vi "SVO.vi"(0 "System no.":i32=1 min=1 max=4 step=1, 2 "Axes to command":string[](array[string]), 3 "Servo mode":bool[](array[boolean]), 5 "error in":errorcluster, 6 "Without axis ID?":bool) -> (19 "error out":errorcluster)   [LabVIEW 2026]
doc: "GCS 3.0\n=====\n\nSVO (Set Servo Mode)\n\nDescription\nSVO sets the mode of operation of the axis by specifying the values 0 or 1 as follows:\n0 -> 0x1 Open-Loop Position\n1 -> 0x2 Closed-Loop Position \nThe mode of operation can only be set when the axis is in the Operation enabled state. For \nfurther details, see \"Drive State Machine\" (p. 101). \n\nFormat\nSVO <AxisID> <Value>\n\nArguments\n<AxisID>\nAn axis of the controller\nThe available axes can be queried with USG? SYS.\nPossible values: Alias of the axis (p. 94) \n<Value>\nValue that sets the mode of operation of the axis\nPossible values:\n0 -> 0x1 Open-Loop Position\n1 -> 0x2 Closed-Loop Position\n\nResponse\nnone\n\nExample\nAxis 1 is to be operated in position control.\n>>svo?\n<<AXIS_1=0\n<<AXIS_2=0\n>>sam?\n<<AXIS_1=0x0\n<<AXIS_2=0x0\n>>svo axis_1 1\n>>svo?\n<<AXIS_1=1\n<<AXIS_2=0\n>>sam?\n<<AXIS_1=0x2\n<<AXIS_2=0x0\n\nNotes\nWith the SVO? command (p. 68), it can be queried whether the current mode of operation is \n0x2.\nThe mode of operation is also displayed in the status register of the axis, which can be queried \nwith the STV? command (p. 66). \nThe SAM command (p. 52) can be used to set all modes of operation supported for the axis.\n\nUser command level\nUSR\n\n\nGCS 2.0\n=====\n\nSets servo-control mode for given axes. If Without axis ID is TRUE, then Axes to command is ignored and first field of Servo mode array is used.\n\nE-516, E-517, E-518: Make sure that all servo switches on the piezo control electronics are set to \"Off\" to give the interface/display module complete control over the servo state.\n\nE-755: Without axis ID = FALSE. When the servo mode is switched off, RNP is automatically performed for the corresponding Nexline channel, which could take a few seconds. Command not available for E-755.101.\n\nE-816: Without axis ID = FALSE. Only one axis per command allowed.\n\nE-861: If you have enabled servo controller is busy for 100 ms, only after this period a next command can be performed.\n\nC-887, F-206, M-8X0: For GCS syntax version = GCS 2.0 or higher (check with CSV?.vi. If CSV?.vi is not supported, syntax version is GCS 1.0), Without axis ID = FALSE. For GCS 1.0, Without axis ID = TRUE and only first field of Servo mode array is valid. \n\nAll other systems: Without axis ID = FALSE"
panel:
  # "SVO (Set Servo Mode)\n\nSVO sets the mode of operation of the axis by specifying the values 0 or 1 as follows:\n0 -> 0x1 Open-Loop Position\n1 -> 0x2 Closed-Loop Position \nThe mode of operation can only be set when the axis is in the Operation enabled state. For \nfurther details, see \"Drive State Machine\"."
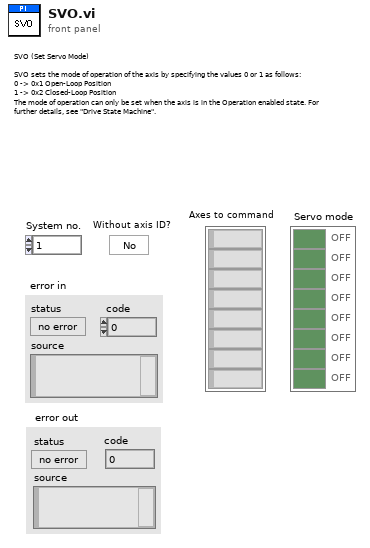
[diagram p1: front panel]
types:
  T1 = typedef "Syntax.ctl" = enum16{"GCS 1.0", "GCS 2.0", "GCS 3.0"}
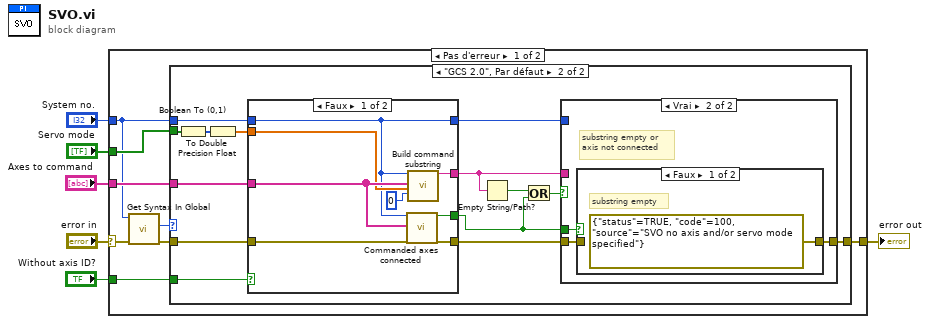
[diagram p0: block diagram]
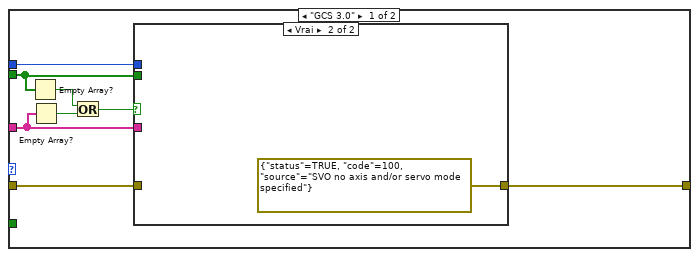
[diagram p2: hidden frame]
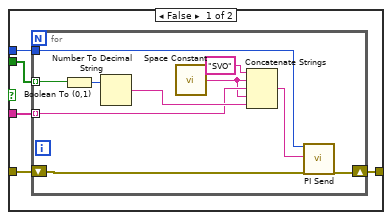
[diagram p3: hidden frame]
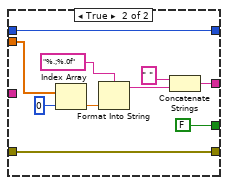
[diagram p4: hidden frame]
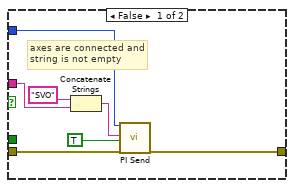
[diagram p5: hidden frame]
diagram:
  n1 = case shown="Pas d'erreur" "error in" {
    selector: "error in" -> [w10 w83]
    tunnel: [w14 w83] -> w6
    tunnel: "System no." -> [w7 _]
    tunnel: "Axes to command" -> [w13 _]
    tunnel: "Servo mode" -> [w12 _]
    tunnel: "Without axis ID?" -> [w11 _]
    frame No Error {
      n2 = call "Get Syntax In Global.vi"("error in"=w10, "System no."=w7) -> ("error out"=w9:errorcluster, "Syntax"=w8:T1)  [unwired: 8 in]
      n3 = case shown="\"GCS 2.0\", Par défaut" w8 {
        tunnel: [w21 w52] -> w14
        tunnel: w13 -> [w19 w50]
        tunnel: w12 -> [w18 w49]
        tunnel: w11 -> [_ w46]
        tunnel: w7 -> [w20 w44]
        tunnel: w9 -> [w22 w45]
        frame "GCS 3.0" {
          n4 = Empty Array?(array=w18) -> (empty?=w16:bool)
          n5 = Empty Array?(array=w19) -> (empty?=w17:bool)
          n6 = Or(x=w16, y=w17) -> (x .or. y?=w15:bool)
          n7 = case shown="Vrai" w15 {
            tunnel: w18 -> [w27 _]
            tunnel: w19 -> [w26 _]
            tunnel: w22 -> [w25 _]
            tunnel: [w24 errorcluster {"status"=TRUE, "code"=100, "source"="SVO no axis and/or servo mode specified"} ("error out")] -> w21
            tunnel: w20 -> [w23 _]
            frame False {
              n8 = for {
                tunnel: w27 -> [w34] mode=indexing
                tunnel: w26 -> [w31] mode=indexing
                shift-right: [w37] -> w24
                shift-left: w25 -> [w36]
                tunnel: w23 -> [w35]
                n9 = Boolean To (0,1)(Boolean=w34) -> (0, 1=w33:i16)
                n10 = Number To Decimal String(number=w33) -> (decimal integer string=w32:string)  [unwired: 1 in]
                n11 = call <vilib>:"Space Constant.vi"() -> ("String"=w30:string)
                n12 = Concatenate Strings("SVO", w30, w31, w30, w32) -> (w28:string)
                n13 = call "PI Send.vi"("System no."=w35, "String to send"=w28, "error in"=w36) -> ("error out"=w37:errorcluster)  [unwired: 3 in, 13 out]
              }
            }
            frame True {
            }
          }
        }
        frame "GCS 2.0", Default {
          n14 = Boolean To (0,1)(Boolean=w49) -> (0, 1=w48:i16[])
          n15 = To Double Precision Float(number=w48) -> (double precision float=w47:dbl[])
          n16 = case shown="Faux" w46 {
            tunnel: [w60 w65] -> w42
            tunnel: w45 -> [w59 w70]
            tunnel: [w58 w70] -> w51
            tunnel: w50 -> [w57 _]
            tunnel: [w56 FALSE] -> w39
            tunnel: w47 -> [w54 w67]
            tunnel: w44 -> [w53 w61]
            tunnel: [w53 w61] -> w43
            frame False {
              n17 = call "Commanded axes connected.vi"("System no."=w53, "Commanded axes"=w57, "error in"=w59) -> ("Controller error"=w56:bool, "error out"=w58:errorcluster)  [unwired: 1 in, 14 out]
              n18 = call "Build command substring.vi"("System no."=w53, "Affected axes"=w57, "Parameters"=w54, "No. of digits"=i16 0 ("No.of digits")) -> ("Command substring"=w60:string)  [unwired: 3 in, 12 out]
            }
            frame True {
              n19 = Index Array(array=w67, index=0 ("Index")) -> (element=w66:dbl)
              n20 = Format Into String(format string="%.;%.0f" ("Format String"), w66) -> (resulting string=w64:string)  [unwired: 2 in, 1 out]
              n21 = Concatenate Strings(" ", w64) -> (w65:string)
            }
          }
          n22 = Empty String/Path?(string/path=w42) -> (empty?=w40:bool)
          n23 = Or(x=w40, y=w39) -> (x .or. y?=w41:bool)
          n24 = case shown="Vrai" w41 {
            tunnel: w42 -> [w76 _]
            tunnel: [w72 w80] -> w52
            tunnel: w51 -> [w73 w78]
            tunnel: w39 -> [_ w79]
            tunnel: w43 -> [w71 _]
            frame False {
              # "axes are connected and\nstring is not empty"
              n25 = Concatenate Strings("SVO", w76) -> (w74:string)
              n26 = call "PI Send.vi"("System no."=w71, "String to send"=w74, "Attach termination char.?"=TRUE ("Attach Linefeed?"), "error in"=w73) -> ("error out"=w72:errorcluster)  [unwired: 2 in, 13 out]
            }
            frame True {
              # "substring empty or \naxis not connected"
              n27 = case shown="Faux" w79 {
                tunnel: [errorcluster {"status"=TRUE, "code"=100, "source"="SVO no axis and/or servo mode specified"} ("error out") w82] -> w80
                tunnel: w78 -> [_ w82]
                frame False {
                  # "substring empty"
                }
                frame True {
                  # "commanded axis\nnot connected"
                }
              }
            }
          }
        }
      }
    }
    frame Error {
    }
  }
  "error out" <- w6
